vi "Page_Info_Read.vi"(6 "ctlReferences":T1, 8 "error in (no error)":errorcluster, 11 "Class in":refnum<class "Installer.lvclass">) -> (0 "error out":errorcluster, 3 "Class out":refnum<class "Installer.lvclass">)   [LabVIEW 2020, in "Installer.lvclass"]
uses:
  <vilib>/AppBuilder/IB_Classes/Installer/Installer.lvclass
  <resource>/Framework/Providers/Builds/Installer/Pages/controls/IB_UI_Page_Info_References.ctl
  <vilib>/AppBuilder/IB_Classes/Installer/Installer.lvclass/Installer.ctl
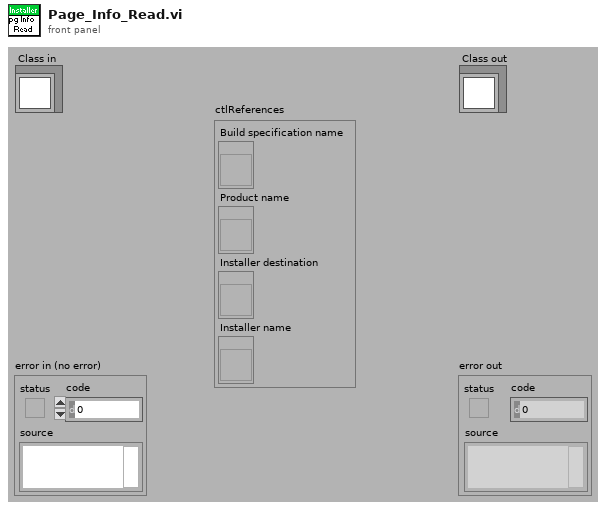
[diagram p1: front panel]
types:
  T1 = typedef "IB_UI_Page_Info_References.ctl" = cluster{"Build specification name":refnum<vi>, "Product name":refnum<vi>, "Installer destination":refnum<vi>, "Installer name":refnum<vi>}
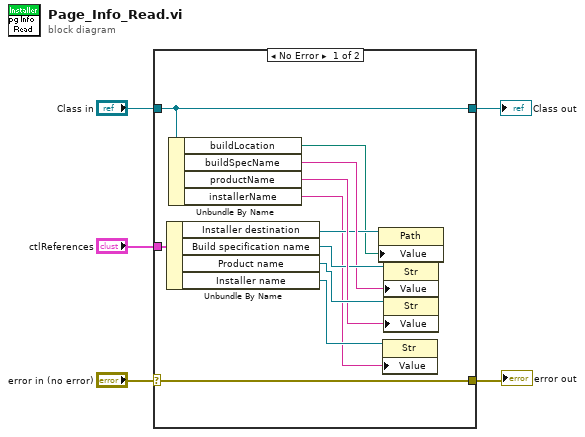
[diagram p0: block diagram]
diagram:
  n1 = case shown="No Error" "error in (no error)" {
    selector: "error in (no error)" -> [w16 w18]
    tunnel: [w16 w18] -> w4
    tunnel: [w15 w17] -> w2
    tunnel: "Class in" -> [w15 w17]
    tunnel: "ctlReferences" -> [w14 _]
    frame No Error {
      n2 = Unbundle By Name(w14) -> ("Installer destination"=w9:refnum<vi>, "Build specification name"=w11:refnum<vi>, "Product name"=w13:refnum<vi>, "Installer name"=w7:refnum<vi>)
      n3 = Unbundle By Name(w15) -> ("buildLocation"=w8:path, "buildSpecName"=w10:string, "productName"=w12:string, "installerName"=w6:string)
      n4 = property class="Path"(reference=w9, "Value"=w8) -> ()  [unwired: 1 in, 2 out]
      n5 = property class="Str"(reference=w7, "Value"=w6) -> ()  [unwired: 1 in, 2 out]
      n6 = property class="Str"(reference=w11, "Value"=w10) -> ()  [unwired: 1 in, 2 out]
      n7 = property class="Str"(reference=w13, "Value"=w12) -> ()  [unwired: 1 in, 2 out]
    }
    frame Error {
    }
  }
  "error out" <- w4
  "Class out" <- w2
